vi "FIFOSettings.vi"(1 "Set/Get":bool, 2 "FIFO Settings(in)":T1={"Measurement"={"Binning (ms)"=1.0, "External Trigger Condition"=0, "Stop Condition:"=2, "Stop Count"=120.0, "Buffer Size (Photons)"=36864, "No of Channels"=2, "Ext Latch Delay"=0}, "ADC"={"Binning (HH)"=0, "Dither Range"=0, "Count Increment"=1, "Mode"=0}, "SYNC"={"SYNC ZC Level (mV)"=10.0, "SYNC Freq Divider"=3, "SYNC Holdoff (ps)"=0.0, "SYNC Threshold (mV)"=20.0}, "TAC"={"TAC Range (ns)"=32.768, "TAC Gain"=1, "TAC Offset (%)"=0.0, "TAC Limit Low (%)"=0.0, "TAC Limit High (%)"=100.0}, "Ch 2"={"Ch2 ZC Level (mV)"=10.0, "Ch2 Holdoff (ps)"=0.0, "Ch2 Threshold (mV)"=20.0}, "Ch 3"={"Ch3 ZC Level (mV)"=10.0, "Ch3 Holdoff (ps)"=0.0, "Ch3 Threshold (mV)"=20.0}, "Ch 4"={"Ch4 ZC Level (mV)"=10.0, "Ch4 Holdoff (ps)"=0.0, "Ch4 Threshold (mV)"=20.0}, "Ch1"={"Ch1 ZC Level (mV)"=10.0, "Ch1 Holdoff (ps)"=0.0, "Ch1 Threshold (mV)"=20.0}} {"Ch1"."Ch1 Threshold (mV)" min=0 max=1000 format="%.2f"; "Ch1"."Ch1 Holdoff (ps)" min=-99999 max=99999 format="%.2f"; "Ch1"."Ch1 ZC Level (mV)" min=0 max=40 format="%.2f"; "Ch 4"."Ch4 Threshold (mV)" min=0 max=1000 format="%.2f"; "Ch 4"."Ch4 Holdoff (ps)" min=-99999 max=99999 format="%.2f"; "Ch 4"."Ch4 ZC Level (mV)" min=0 max=40 format="%.2f"; "Ch 3"."Ch3 Threshold (mV)" min=0 max=1000 format="%.2f"; "Ch 3"."Ch3 Holdoff (ps)" min=-99999 max=99999 format="%.2f"; "Ch 3"."Ch3 ZC Level (mV)" min=0 max=40 format="%.2f"; "Ch 2"."Ch2 Threshold (mV)" min=0 max=1000 format="%.2f"; "Ch 2"."Ch2 Holdoff (ps)" min=-99999 max=99999 format="%.2f"; "Ch 2"."Ch2 ZC Level (mV)" min=0 max=40 format="%.2f"; "TAC"."TAC Limit High (%)" min=0 max=100 format="%.2f"; "TAC"."TAC Limit Low (%)" min=0 max=100 format="%.2f"; "TAC"."TAC Offset (%)" min=0 max=100 format="%.2f"; "TAC"."TAC Gain" min=1 max=15 step=1; "TAC"."TAC Range (ns)" min=0 max=2000 format="%.2f"; "SYNC"."SYNC Threshold (mV)" min=0 max=1000 format="%.2f"; "SYNC"."SYNC Holdoff (ps)" min=-99999 max=99999 format="%.2f"; "SYNC"."SYNC Freq Divider" items=["1", "2", "4", "8", "16"]; "SYNC"."SYNC ZC Level (mV)" min=0 max=40 format="%.2f"; "ADC"."Mode" items=["T3"]; "ADC"."Binning (HH)" items=["1", "2", "4", "8", "16", "32", "64", "128", "256", "512", "1024"]; "ADC"."Count Increment" min=1 max=255 step=1; "ADC"."Dither Range" min=0 max=256 step=32; "Measurement"."Ext Latch Delay" min=0 max=255 step=1; "Measurement"."Buffer Size (Photons)" min=512 step=512; "Measurement"."Stop Count" format="%.2f"; "Measurement"."Stop Condition:" items=["None", "Photon Count", "Time (s)"]; "Measurement"."External Trigger Condition" max=2 step=1; "Measurement"."No of Channels" max=14; "Measurement"."Binning (ms)" min=1e-07 max=100000 format="%.3f"}) -> (0 "FIFO Settings(out)":T1={"Measurement"={"Binning (ms)"=1.0, "External Trigger Condition"=0, "Stop Condition:"=2, "Stop Count"=120.0, "Buffer Size (Photons)"=10240, "No of Channels"=1, "Ext Latch Delay"=0}, "ADC"={"Binning (HH)"=0, "Dither Range"=0, "Count Increment"=1, "Mode"=0}, "SYNC"={"SYNC ZC Level (mV)"=10.0, "SYNC Freq Divider"=3, "SYNC Holdoff (ps)"=0.0, "SYNC Threshold (mV)"=20.0}, "TAC"={"TAC Range (ns)"=32.765, "TAC Gain"=1, "TAC Offset (%)"=0.0, "TAC Limit Low (%)"=0.0, "TAC Limit High (%)"=100.0}, "Ch 2"={"Ch2 ZC Level (mV)"=10.0, "Ch2 Holdoff (ps)"=0.0, "Ch2 Threshold (mV)"=20.0}, "Ch 3"={"Ch3 ZC Level (mV)"=10.0, "Ch3 Holdoff (ps)"=0.0, "Ch3 Threshold (mV)"=20.0}, "Ch 4"={"Ch4 ZC Level (mV)"=10.0, "Ch4 Holdoff (ps)"=0.0, "Ch4 Threshold (mV)"=20.0}, "Ch1"={"Ch1 ZC Level (mV)"=10.0, "Ch1 Holdoff (ps)"=0.0, "Ch1 Threshold (mV)"=20.0}} {"Ch1"."Ch1 Threshold (mV)" min=0 max=1000 format="%.2f"; "Ch1"."Ch1 Holdoff (ps)" min=-99999 max=99999 format="%.2f"; "Ch1"."Ch1 ZC Level (mV)" min=0 max=40 format="%.2f"; "Ch 4"."Ch4 Threshold (mV)" min=0 max=1000 format="%.2f"; "Ch 4"."Ch4 Holdoff (ps)" min=-99999 max=99999 format="%.2f"; "Ch 4"."Ch4 ZC Level (mV)" min=0 max=40 format="%.2f"; "Ch 3"."Ch3 Threshold (mV)" min=0 max=1000 format="%.2f"; "Ch 3"."Ch3 Holdoff (ps)" min=-99999 max=99999 format="%.2f"; "Ch 3"."Ch3 ZC Level (mV)" min=0 max=40 format="%.2f"; "Ch 2"."Ch2 Threshold (mV)" min=0 max=1000 format="%.2f"; "Ch 2"."Ch2 Holdoff (ps)" min=-99999 max=99999 format="%.2f"; "Ch 2"."Ch2 ZC Level (mV)" min=0 max=40 format="%.2f"; "TAC"."TAC Limit High (%)" min=0 max=100 format="%.2f"; "TAC"."TAC Limit Low (%)" min=0 max=100 format="%.2f"; "TAC"."TAC Offset (%)" min=0 max=100 format="%.2f"; "TAC"."TAC Gain" min=1 max=15 step=1; "TAC"."TAC Range (ns)" min=50 max=2000 format="%.2f"; "SYNC"."SYNC Threshold (mV)" min=0 max=1000 format="%.2f"; "SYNC"."SYNC Holdoff (ps)" min=-99999 max=99999 format="%.2f"; "SYNC"."SYNC Freq Divider" items=["1", "2", "4", "8", "16"]; "SYNC"."SYNC ZC Level (mV)" min=0 max=40 format="%.2f"; "ADC"."Mode" items=["T3"]; "ADC"."Binning (HH)" items=["1", "2", "4", "8", "16", "32", "64", "128", "256", "512", "1024"]; "ADC"."Count Increment" min=1 max=255 step=1; "ADC"."Dither Range" min=0 max=256 step=32; "Measurement"."Ext Latch Delay" min=0 max=255 step=1; "Measurement"."Buffer Size (Photons)" min=512 step=512; "Measurement"."Stop Count" format="%.2f"; "Measurement"."Stop Condition:" items=["None", "Photon Count", "Time (s)"]; "Measurement"."External Trigger Condition" max=2 step=1; "Measurement"."No of Channels" max=14; "Measurement"."Binning (ms)" min=1e-07 max=100000 format="%.3f"})   [LabVIEW 2009]
uses:
  FIFOSettings.ctt
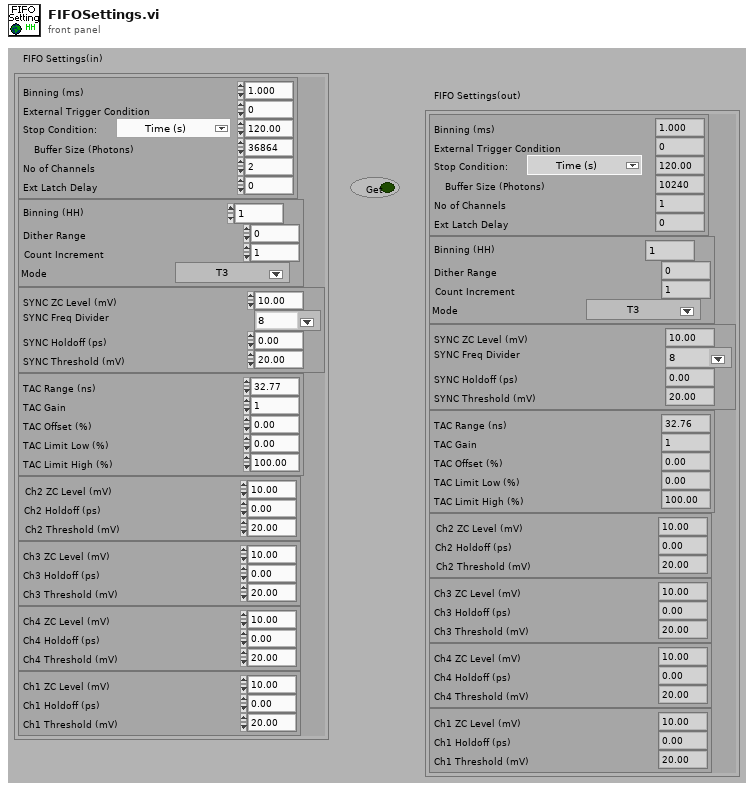
[diagram p1: front panel]
types:
  T1 = typedef "FIFOSettings.ctt" = cluster{"Measurement":cluster{"Binning (ms)":sgl, "External Trigger Condition":u16, "Stop Condition:":u16, "Stop Count":dbl, "Buffer Size (Photons)":u32, "No of Channels":u16, "Ext Latch Delay":i16}, "ADC":cluster{"Binning (HH)":i16, "Dither Range":i16, "Count Increment":i16, "Mode":u16}, "SYNC":cluster{"SYNC ZC Level (mV)":sgl, "SYNC Freq Divider":u16, "SYNC Holdoff (ps)":sgl, "SYNC Threshold (mV)":sgl}, "TAC":cluster{"TAC Range (ns)":sgl, "TAC Gain":i16, "TAC Offset (%)":sgl, "TAC Limit Low (%)":sgl, "TAC Limit High (%)":sgl}, "Ch 2":cluster{"Ch2 ZC Level (mV)":sgl, "Ch2 Holdoff (ps)":sgl, "Ch2 Threshold (mV)":sgl}, "Ch 3":cluster{"Ch3 ZC Level (mV)":sgl, "Ch3 Holdoff (ps)":sgl, "Ch3 Threshold (mV)":sgl}, "Ch 4":cluster{"Ch4 ZC Level (mV)":sgl, "Ch4 Holdoff (ps)":sgl, "Ch4 Threshold (mV)":sgl}, "Ch1":cluster{"Ch1 ZC Level (mV)":sgl, "Ch1 Holdoff (ps)":sgl, "Ch1 Threshold (mV)":sgl}}
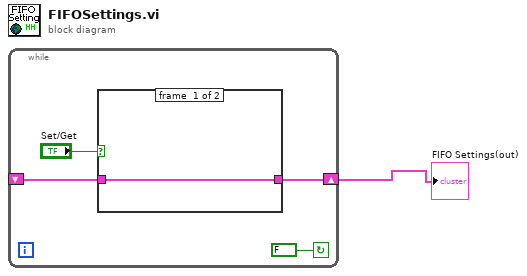
[diagram p0: block diagram]
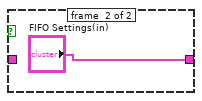
[diagram p2: hidden frame]
diagram:
  n1 = while {
    shift-right: [w2] -> w1
    shift-left: _ -> [w3]
    stop <- FALSE continue-if-true
    n2 = case shown="True" "Set/Get" {
      tunnel: [w6 "FIFO Settings(in)"] -> w2
      tunnel: w3 -> [w6 _]
      frame #0 {
      }
      frame #1 {
      }
    }
  }
  "FIFO Settings(out)" <- w1
